vi "Double Exponential Guess Parameters.vi"(10 "Y":dbl[](array[numeric]), 11 "X":dbl[](array[numeric])) -> (1 "2-Exp Guess Parameters":dbl[](array[numeric]))   [LabVIEW 2019]
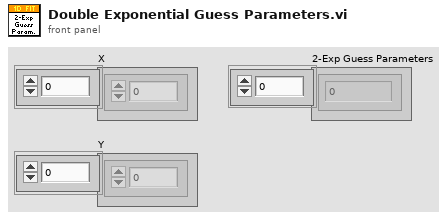
[diagram p1: front panel]
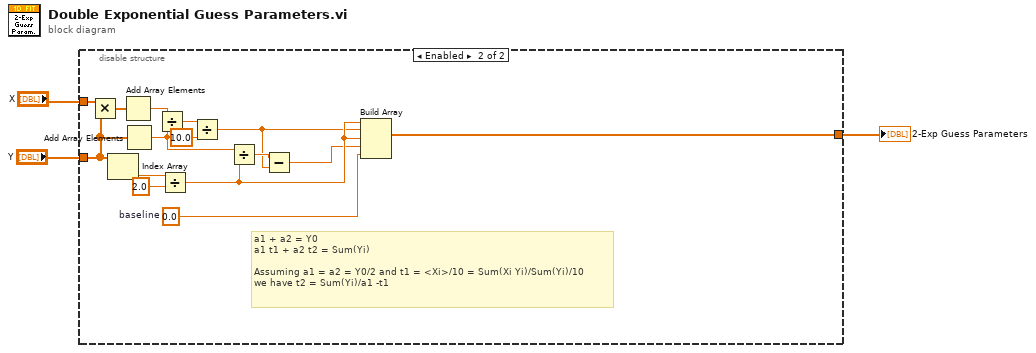
[diagram p0: block diagram]
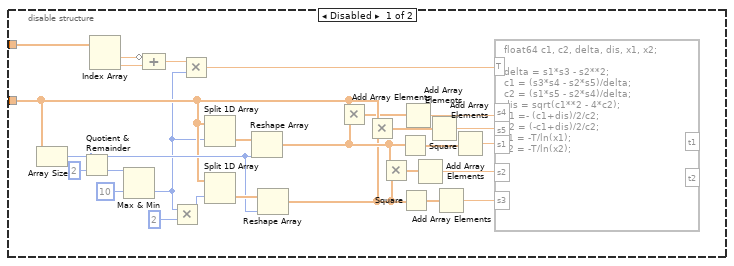
[diagram p2: hidden frame]
diagram:
  n1 = disable-structure shown="Enabled" {
    disable-tunnel: "X" -> [w30 w43]
    disable-tunnel: "Y" -> [w20 w41]
    disable-tunnel: [_ w32] -> w1
    frame Disabled {
      n2 = Array Size(array=w20) -> (size(s)=w21:i32)
      n3 = Quotient & Remainder(x=w21, y=2) -> (floor(x/y)=w26:i32)  [unwired: 1 out]
      n4 = Index Array(array=w30) -> (element #1=w29:dbl, element #2=w28:dbl)  [unwired: 2 in]
      n5 = Max & Min(x=w26, y=10) -> (min(x,y)=w6:i32)  [unwired: 1 out]
      n6 = Compound Arithmetic op=ADD(invert w29, w28) -> (w7:dbl)
      n7 = Multiply(x=w6, y=2) -> (x*y=w24:i32)
      n8 = Multiply(x=w7, y=w6) -> (x*y=w5:dbl)
      n9 = Split 1D Array(array=w20, index=w6) -> (second subarray=w23:dbl[])  [unwired: 1 out]
      n10 = Split 1D Array(array=w20, index=w24) -> (second subarray=w22:dbl[])  [unwired: 1 out]
      n11 = Reshape Array(w23, w21) -> (w19:dbl[])
      n12 = Reshape Array(w22, w21) -> (w18:dbl[])
      n13 = Multiply(x=w20, y=w19) -> (x*y=w17:dbl[])
      n14 = Multiply(x=w20, y=w18) -> (x*y=w16:dbl[])
      n15 = Multiply(x=w19, y=w18) -> (x*y=w14:dbl[])
      n16 = Square(x=w19) -> (x^2=w15:dbl[])
      n17 = Square(x=w18) -> (x^2=w13:dbl[])
      n18 = Add Array Elements(numeric array=w17) -> (sum=w12:dbl)
      n19 = Add Array Elements(numeric array=w14) -> (sum=w9:dbl)
      n20 = Add Array Elements(numeric array=w16) -> (sum=w11:dbl)
      n21 = Add Array Elements(numeric array=w13) -> (sum=w8:dbl)
      n22 = Add Array Elements(numeric array=w15) -> (sum=w10:dbl)
      n23 = formula code="float64 c1, c2, delta, dis, x1, x2;\n\ndelta = s1*s3 - s2**2;\nc1 = (s3*s4 - s2*s5)/delta;\nc2 = (s1*s5 - s2*s4)/delta;\ndis = sqrt(c1**2 - 4*c2);\nx1 =- (c1+dis)/2/c2;\nx2 = (-c1+dis)/2/c2; \nt1 = -T/ln(x1);\nt2 = -T/ln(x2);"("s4"=w12, "s5"=w11, "s1"=w10, "s2"=w9, "s3"=w8, "T"=w5) -> ()  [unwired: 2 out]
    }
    frame Enabled {
      w31 = 0.0  # baseline
      # "a1 + a2 = Y0\na1 t1 + a2 t2 = Sum(Yi)\n\nAssuming a1 = a2 = Y0/2 and t1 = <Xi>/10 = Sum(Xi Yi)/Sum(Yi)/10\nwe have t2 = Sum(Yi)/a1 -t1"
      n24 = Multiply(x=w43, y=w41) -> (x*y=w42:dbl[])
      n25 = Index Array(array=w41) -> (element=w45:dbl)  [unwired: 1 in]
      n26 = Add Array Elements(numeric array=w42) -> (sum=w40:dbl)
      n27 = Add Array Elements(numeric array=w41) -> (sum=w37:dbl)
      n28 = Divide(x=w40, y=w37) -> (x/y=w39:dbl)
      n29 = Divide(x=w45, y=2.0) -> (x/y=w36:dbl)
      n30 = Divide(x=w39, y=10.0) -> (x/y=w34:dbl)
      n31 = Divide(x=w37, y=w36) -> (x/y=w35:dbl)
      n32 = Subtract(x=w35, y=w34) -> (x-y=w33:dbl)
      n33 = Build Array(w36, w34, w36, w33, w31) -> (w32:dbl[])
    }
  }
  "2-Exp Guess Parameters" <- w1
